vi "Write Binary.vi"(6 "error in (no error)":errorcluster, 7 "Bytes":u8[](array[numeric]), 8 "timeout ms (1000)":i32=1000, 9 "Websocket Handler in":refnum<class "Websocket Handler.lvclass">) -> (0 "error out":errorcluster, 3 "Websocket Handler out":refnum<class "Websocket Handler.lvclass">)   [LabVIEW 2020, in "wamplv.lvlib" / "Websocket Handler.lvclass"]
uses:
  Websocket Handler.lvclass
  Websocket Handler.lvclass/Websocket Handler.ctl
  <vilib>/MediaMongrels Ltd/WebSockets/WebSockets/WebSocket Client/WebSocket Client.lvclass
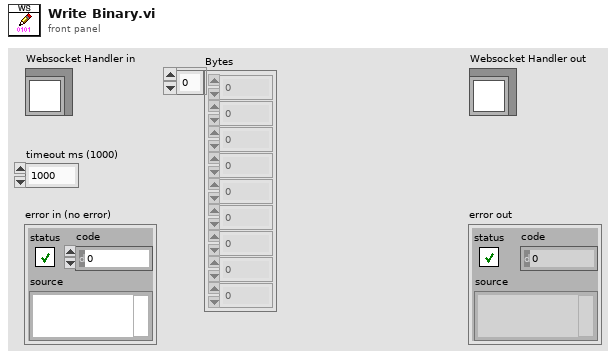
[diagram p1: front panel]
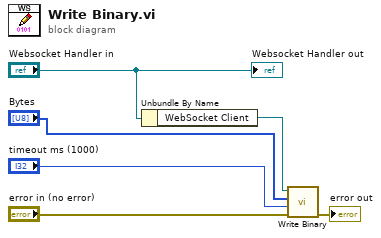
[diagram p0: block diagram]
diagram:
  n1 = Unbundle By Name("Websocket Handler in") -> ("WebSocket Client"=w6:refnum<class "WebSocket Client.lvclass">)
  n2 = call-dynamic "Write Binary.vi"("error in (no error)"="error in (no error)", "timeout ms (5000)"="timeout ms (1000)", "Binary Data"="Bytes", "WebSocket in"=w6) -> ("error out"=→"error out":errorcluster)  [unwired: 6 in, 1 out]
  "Websocket Handler out" <- "Websocket Handler in"
